vi "Controller.vi"() -> ()   [LabVIEW 2012]
uses:
  <vilib>/Instr/_visa.llb/VISA Flush IO Buffer Mask.ctl
  <vilib>/Instr/_visa.llb/VISA Configure Serial Port (Instr).vi
panel:
  out "Waveform Chart":i32(graph)
  in  "Hexadecimal Input String":string
  in  "Stop":bool
  in  "UART configuration":enum32{"Basic", "Advanced"}(tab)
  in  "Port name":refnum<visa-resource-name>
  in  "Baud rate":T1(ring)
  in  "Data bits":u16=8 min=5 max=8 step=1
  in  "Stop bits":u16(ring)=10 items=["1.0"=10, "1.5"=15, "2.0"=20]
  in  "parity (0:none)":enum16{"None", "Odd", "Even", "Mark", "Space"}(ring)
  in  "Loop wait [ms]":u32
  in  "Waiting time [ms]":u32
  in  "Timeout [ms]":u32=10000
  in  "Flow control":u16(ring) items=["None", "XON/XOFF", "RTS/CTS", "XON/XOFF & RTS/CTS", "DTR/DSR", "XON/XOFF & DTR/DSR"]
  in  "Termination char\n(0xA = '\\n' = LF)":u8=10 format="%.0x"
  in  "Enable Termination\nChar (T)":bool=TRUE
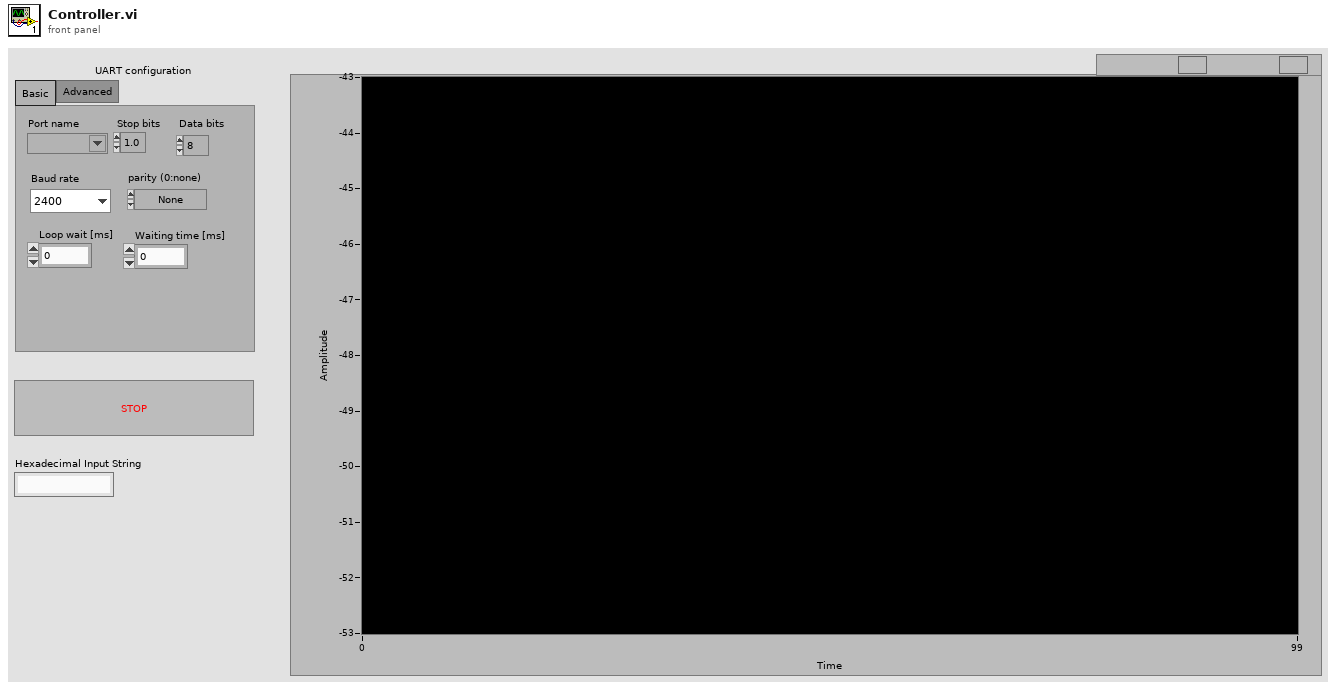
[diagram p1: front panel]
types:
  T1 = enum16{"2400\n", "4800", "9600\n", "19200", "38400", "57600", "115200"}
  T2 = typedef "VISA Flush IO Buffer Mask.ctl" = u16
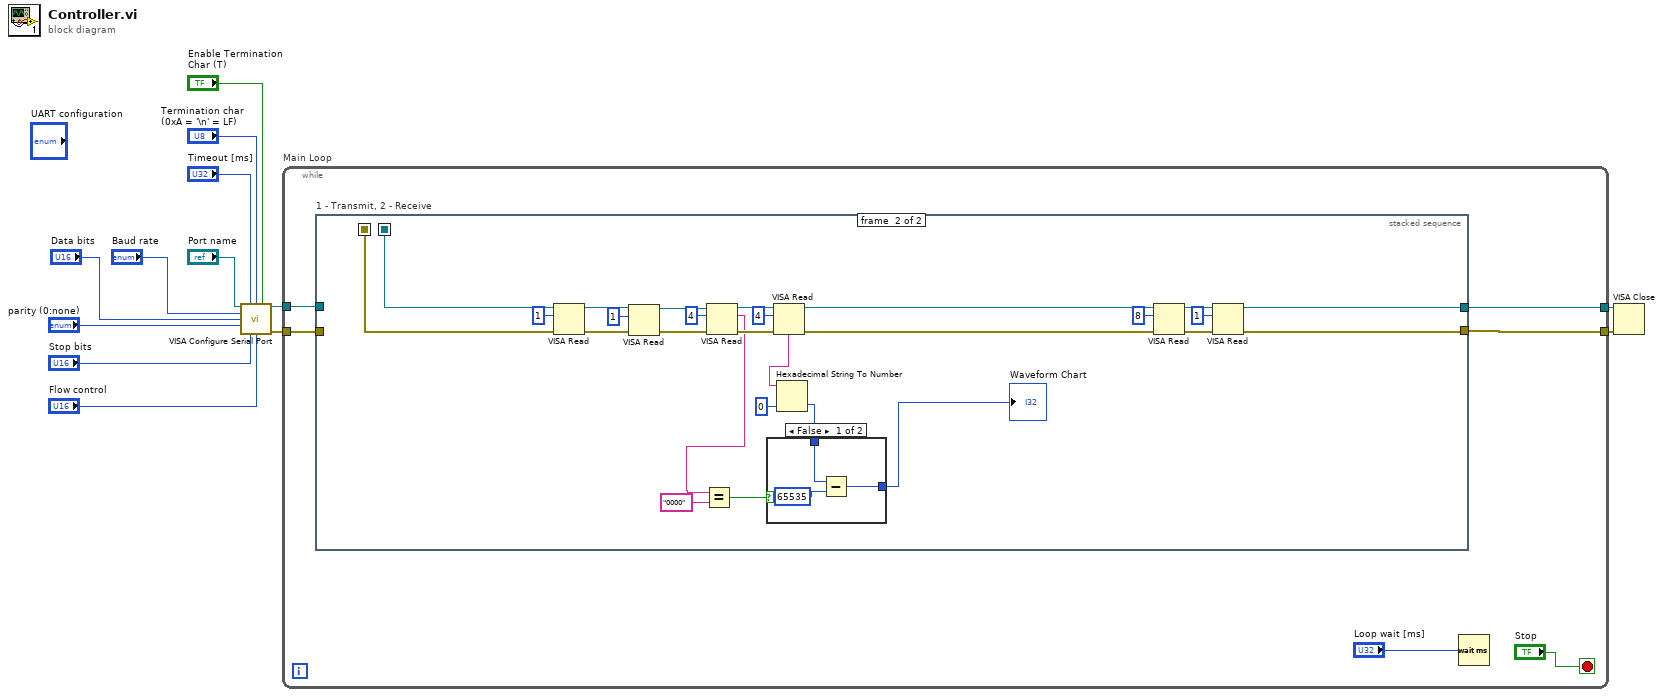
[diagram p0: block diagram]
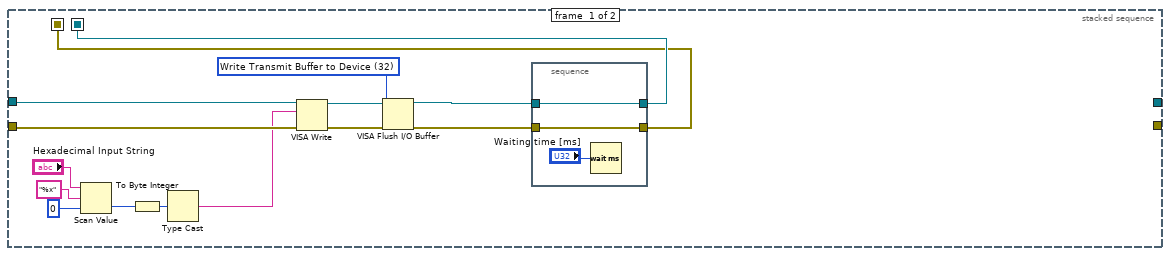
[diagram p2: hidden frame]
diagram:
  n1 = call-poly "VISA Configure Serial Port"("VISA resource name"="Port name", "timeout (10sec)"="Timeout [ms]", "termination char\n(0xA = '\\n' = LF)"="Termination char\n(0xA = '\\n' = LF)", "Enable Termination\nChar (T)"="Enable Termination\nChar (T)", "baud rate (9600)"="Baud rate", "data bits (8)"="Data bits", "parity (0:none)"="parity (0:none)", "stop bits (10: 1 bit)"="Stop bits", "flow control (0:none)"="Flow control") -> ("VISA resource name out"=w4:refnum<visa-resource-name>, "error out"=w3:errorcluster)  [unwired: 5 in]
  n2 = while "Main Loop" {
    tunnel: w4 -> [w19]
    tunnel: w3 -> [w18]
    tunnel: [w14] -> w2
    tunnel: [w15] -> w1
    stop <- "Stop" stop-if-true
    n3 = stacked-sequence "1 - Transmit, 2 - Receive" {
      seq-local: [w29 _] -> [_ w38]
      seq-local: [w28 _] -> [_ w39]
      tunnel: w19 -> [w31 _]
      tunnel: w18 -> [w30 _]
      tunnel: [_ w55] -> w15
      tunnel: [_ w54] -> w14
      frame #0 {
        w32 = T2 32 items=["Flush Receive Buffer"=16, "Write Transmit Buffer to Device"=32, "Flush Receive Buffer (No I/O)"=64, "Flush Transmit Buffer"=128] ("Mask")
        n4 = Scan Value(string="Hexadecimal Input String", format string="%x", default (0 dbl)=0) -> (value=w23:i32)  [unwired: 1 out]
        n5 = To Byte Integer(number=w23) -> (8bit integer=w22:i8)
        n6 = Type Cast(x=w22) -> (*(type *) &x=w24:string)  [unwired: 1 in]
        n7 = VISA Write(VISA resource name=w31, write buffer=w24, error in (no error)=w30) -> (VISA resource name out=w33:refnum<visa-resource-name>, error out=w34:errorcluster)  [unwired: 1 out]
        n8 = VISA Flush I/O Buffer(VISA resource name=w33, mask (16)=w32, error in (no error)=w34) -> (VISA resource name out=w20:refnum<visa-resource-name>, error out=w21:errorcluster)
        n9 = stacked-sequence "Waiting time" {
          tunnel: [w36] -> w29
          tunnel: w20 -> [w36]
          tunnel: [w35] -> w28
          tunnel: w21 -> [w35]
          frame #0 {
            n10 = Wait (ms)(milliseconds to wait="Waiting time [ms]") -> ()  [unwired: 1 out]
          }
        }
      }
      frame #1 {
        n11 = VISA Read(VISA resource name=w38, byte count=u32 1, error in (no error)=w39) -> (VISA resource name out=w63:refnum<visa-resource-name>, error out=w62:errorcluster)  [unwired: 2 out]
        n12 = VISA Read(VISA resource name=w63, byte count=u32 1, error in (no error)=w62) -> (VISA resource name out=w52:refnum<visa-resource-name>, error out=w48:errorcluster)  [unwired: 2 out]
        n13 = VISA Read(VISA resource name=w52, byte count=u32 4, error in (no error)=w48) -> (VISA resource name out=w51:refnum<visa-resource-name>, read buffer=w42:string, error out=w49:errorcluster)  [unwired: 1 out]
        n14 = Equal?(x=w42, y="0000") -> (x = y?=w41:bool)
        n15 = VISA Read(VISA resource name=w51, byte count=u32 4, error in (no error)=w49) -> (VISA resource name out=w60:refnum<visa-resource-name>, read buffer=w46:string, error out=w59:errorcluster)  [unwired: 1 out]
        n16 = Hexadecimal String To Number(string=w46, default (0uL)=0 ("default (0 U32)")) -> (number=w44:i32)  [unwired: 1 in, 1 out]
        n17 = case shown="False" w41 {
          tunnel: w44 -> [w66 w68]
          tunnel: [w67 w68] -> w40
          frame False {
            n18 = Subtract(x=w66, y=65535) -> (x-y=w67:i32)
          }
          frame True {
          }
        }
        "Waveform Chart" <- w40
        n19 = VISA Read(VISA resource name=w60, byte count=u32 8, error in (no error)=w59) -> (VISA resource name out=w57:refnum<visa-resource-name>, error out=w56:errorcluster)  [unwired: 2 out]
        n20 = VISA Read(VISA resource name=w57, byte count=u32 1, error in (no error)=w56) -> (VISA resource name out=w54:refnum<visa-resource-name>, error out=w55:errorcluster)  [unwired: 2 out]
      }
    }
    n21 = Wait (ms)(milliseconds to wait="Loop wait [ms]") -> ()  [unwired: 1 out]
  }
  n22 = VISA Close(VISA resource name=w2, error in (no error)=w1) -> ()  [unwired: 1 out]
